vi "Configure Measurements (Inrush).vi"(8 "error in (no error)":errorcluster, 9 "Current Range (100Apk)":i32(ring)=5 items=["0.1Apk", "0.4Apk", "1.6Apk", "6.25Apk", "25Apk", "100Apk"], 10 "Inrush Measurements":i32[](listbox)=[2, 3, 4, 5], 11 "VISA resource name":refnum<visa-resource-name>) -> (0 "error out":errorcluster, 3 "VISA resource name out":refnum<visa-resource-name>)   [LabVIEW 2015, in "Voltech PM1000+.lvlib"]
doc: "Configures the measurement itmes, and return the selected measurement list and indicators. This vi is used when PM1000+ is set to Inrush mode by using \"Configure Mode\" vi."
uses:
  <instrlib>/Voltech PM1000+/Voltech PM1000+.lvlib
panel:
  # "Notice:  \nHold \"Ctrl\" key and click the \nmeasurements to select \nmultiple items."
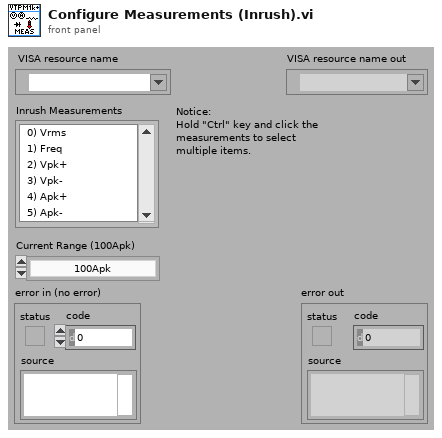
[diagram p1: front panel]
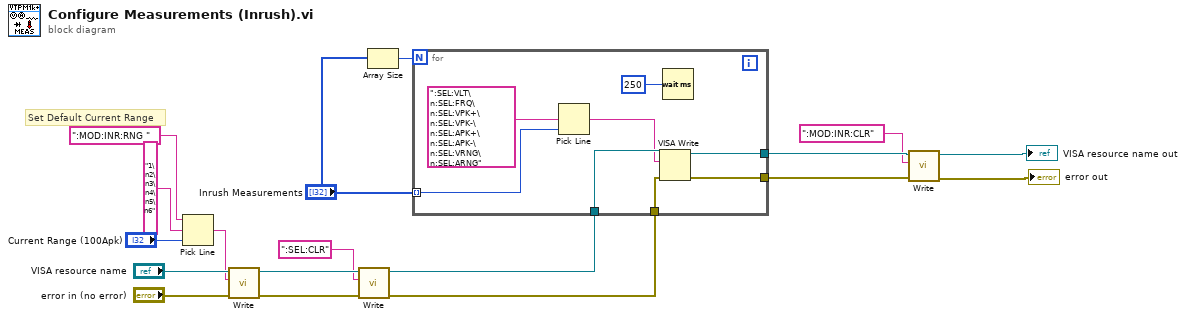
[diagram p0: block diagram]
diagram:
  # "Set Default Current Range"
  n1 = Pick Line(string ("")=":MOD:INR:RNG " ("write buffer"), multi-line string="1\n2\n3\n4\n5\n6", line index="Current Range (100Apk)") -> (output string=w5:string)
  n2 = call <instrlib>:"Write.vi"("error in (no error)"="error in (no error)", "Write Buffer"=w5, "VISA resource name"="VISA resource name") -> ("error out"=w10:errorcluster, "VISA resource name out"=w11:refnum<visa-resource-name>)  [unwired: 7 in]
  n3 = call <instrlib>:"Write.vi"("error in (no error)"=w10, "Write Buffer"=":SEL:CLR" ("multi-line string"), "VISA resource name"=w11) -> ("error out"=w12:errorcluster, "VISA resource name out"=w13:refnum<visa-resource-name>)  [unwired: 7 in]
  n4 = Array Size(array="Inrush Measurements") -> (size(s)=w15:i32)
  n5 = for {
    N: w15 -> [_]
    tunnel: "Inrush Measurements" -> [w25] mode=indexing
    tunnel: w13 -> [w23]
    tunnel: w12 -> [w22]
    tunnel: [w21] -> w7
    tunnel: [w20] -> w6
    n6 = Pick Line(multi-line string=":SEL:VLT\n:SEL:FRQ\n:SEL:VPK+\n:SEL:VPK-\n:SEL:APK+\n:SEL:APK-\n:SEL:VRNG\n:SEL:ARNG", line index=w25) -> (output string=w19:string)  [unwired: 1 in]
    n7 = VISA Write(VISA resource name=w23, write buffer=w19, error in (no error)=w22) -> (VISA resource name out=w21:refnum<visa-resource-name>, error out=w20:errorcluster)  [unwired: 1 out]
    n8 = Wait (ms)(milliseconds to wait=250) -> ()  [unwired: 1 out]
  }
  n9 = call <instrlib>:"Write.vi"("error in (no error)"=w6, "Write Buffer"=":MOD:INR:CLR", "VISA resource name"=w7) -> ("error out"=→"error out":errorcluster, "VISA resource name out"=→"VISA resource name out":refnum<visa-resource-name>)  [unwired: 7 in]
